vi "Unflatten Dependencies From String Array.vi"(3 "Flattened Dependencies":string[][](array[string])) -> (0 "Deps":T1[](array[typedef]), 1 "User Deps":T2[](array[typedef]))   [LabVIEW 2020, in "LMH-Toolbox.lvlib" / "LMH-Installer Tools.lvlib"]
uses:
  LMH-Installer Tools.lvlib
  Type Defs/User Dependency.ctl
  Type Defs/Dependecy.ctl
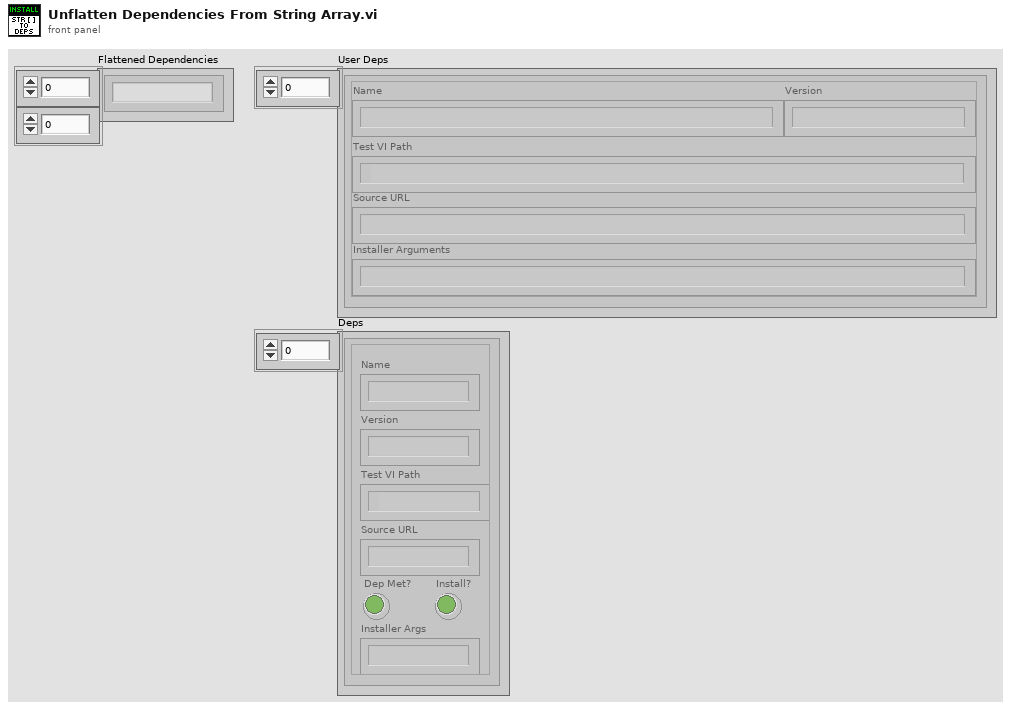
[diagram p1: front panel]
types:
  T1 = typedef "LMH-Toolbox.lvlib/LMH-Installer Tools.lvlib/Dependecy.ctl" = cluster{"Name":string, "Version":string, "Test VI Path":path, "Source URL":string, "Dep Met?":bool, "Install?":bool, "Installer Args":string}
  T2 = typedef "LMH-Toolbox.lvlib/LMH-Installer Tools.lvlib/User Dependency.ctl" = cluster{"Name":string, "Version":string, "Test VI Path":path, "Source URL":string, "Installer Arguments":string}
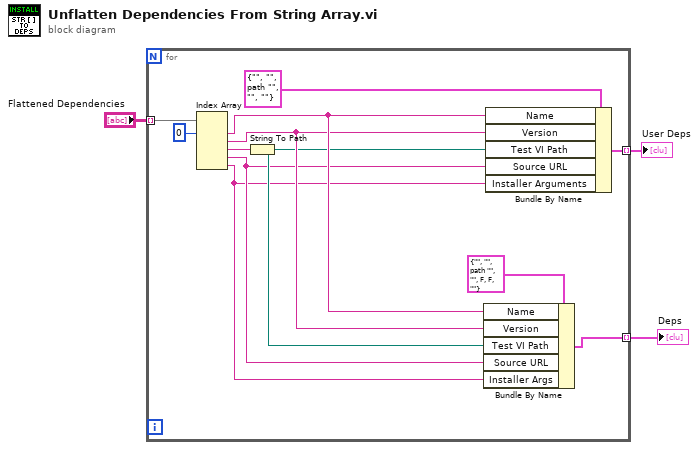
[diagram p0: block diagram]
diagram:
  n1 = for {
    tunnel: "Flattened Dependencies" -> [w15] mode=indexing
    tunnel: [w13] -> w2 mode=indexing
    tunnel: [w6] -> w1 mode=indexing
    n2 = Index Array(array=w15, index #1=0 ("index")) -> (element #1=w10:string, element #2=w9:string, element #3=w4:string, element #4=w7:string, element #5=w5:string)  [unwired: 4 in]
    n3 = String To Path(string=w4) -> (path=w8:path)
    n4 = Bundle By Name(cluster=T1 {"Name"="", "Version"="", "Test VI Path"=path "", "Source URL"="", "Dep Met?"=FALSE, "Install?"=FALSE, "Installer Args"=""} ("Dependecy"), "Name"=w10, "Version"=w9, "Test VI Path"=w8, "Source URL"=w7, "Installer Args"=w5) -> (w6:T1)
    n5 = Bundle By Name(cluster=T2 {"Name"="", "Version"="", "Test VI Path"=path "", "Source URL"="", "Installer Arguments"=""} ("User Dependency"), "Name"=w10, "Version"=w9, "Test VI Path"=w8, "Source URL"=w7, "Installer Arguments"=w5) -> (w13:T2)
  }
  "User Deps" <- w2
  "Deps" <- w1
